vi "Filter Negative Numbers.vi"(4 "Numeric In":i32) -> (1 "Numeric Out":i32)   [LabVIEW 2014]
doc: "Coerce negative numbers to 0."
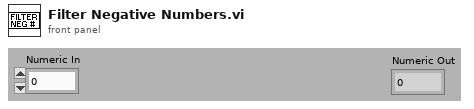
[diagram p1: front panel]
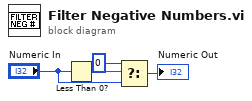
[diagram p0: block diagram]
diagram:
  n1 = Less Than 0?(x="Numeric In") -> (x < 0?=w4:bool)
  n2 = Select(t=0, s=w4, f="Numeric In") -> (s? t:f=→"Numeric Out":i32)
